vi "find and draw circles.vi"(0 "Image Src":T1, 1 "module path":path, 2 "function name":string="get_circels", 3 "initialized array":dbl[][](array[numeric]), 4 "Image Dst":T1, 5 "error in (no error)":errorcluster, 6 "session in":refnum<k35>, 7 "Run/Stop":bool, 8 "grading Thr":dbl[](array[numeric]), 9 "bias":i8=14) -> (14 "session out":refnum<k35>, 15 "circle info":dbl[][](array[numeric]), 16 "Image Out":T1, 18 "error out":errorcluster, 19 "pellet detected?":bool)   [LabVIEW 2019]
uses:
  <vilib>/vision/Image Controls.llb/IMAQ Image.ctl
  <vilib>/Utility/error.llb/DialogType.ctl
  detectedPellet.lvlib
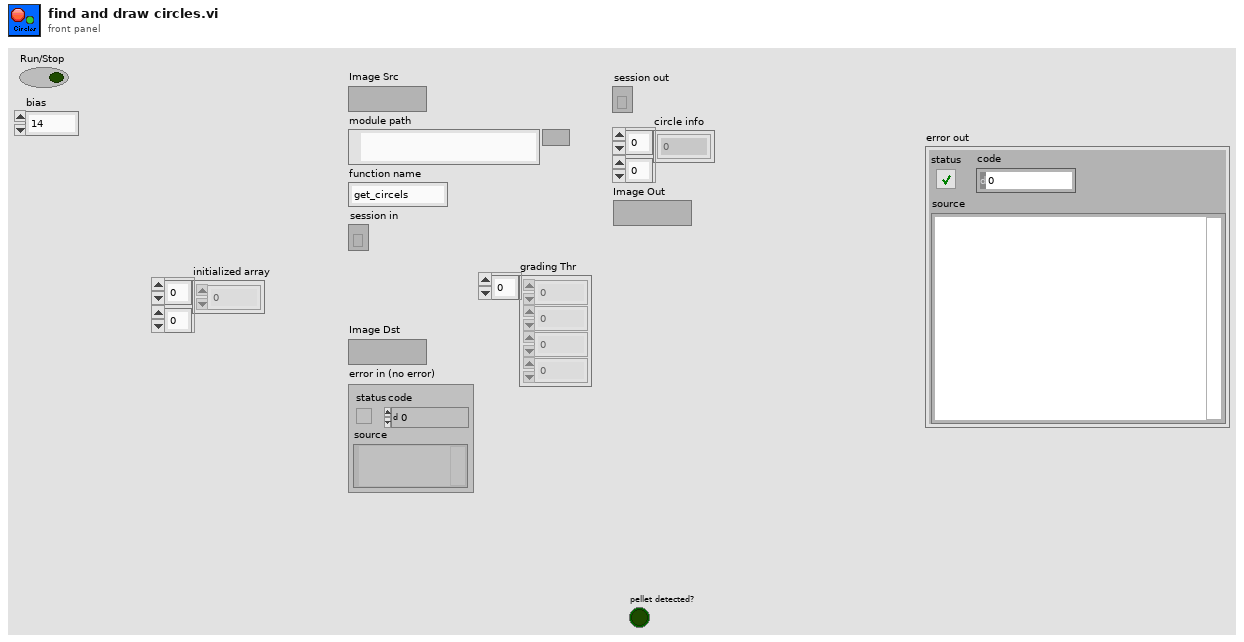
[diagram p1: front panel]
types:
  T1 = typedef "IMAQ Image.ctl" = refnum<image>
  T2 = typedef "DialogType.ctl" = u16
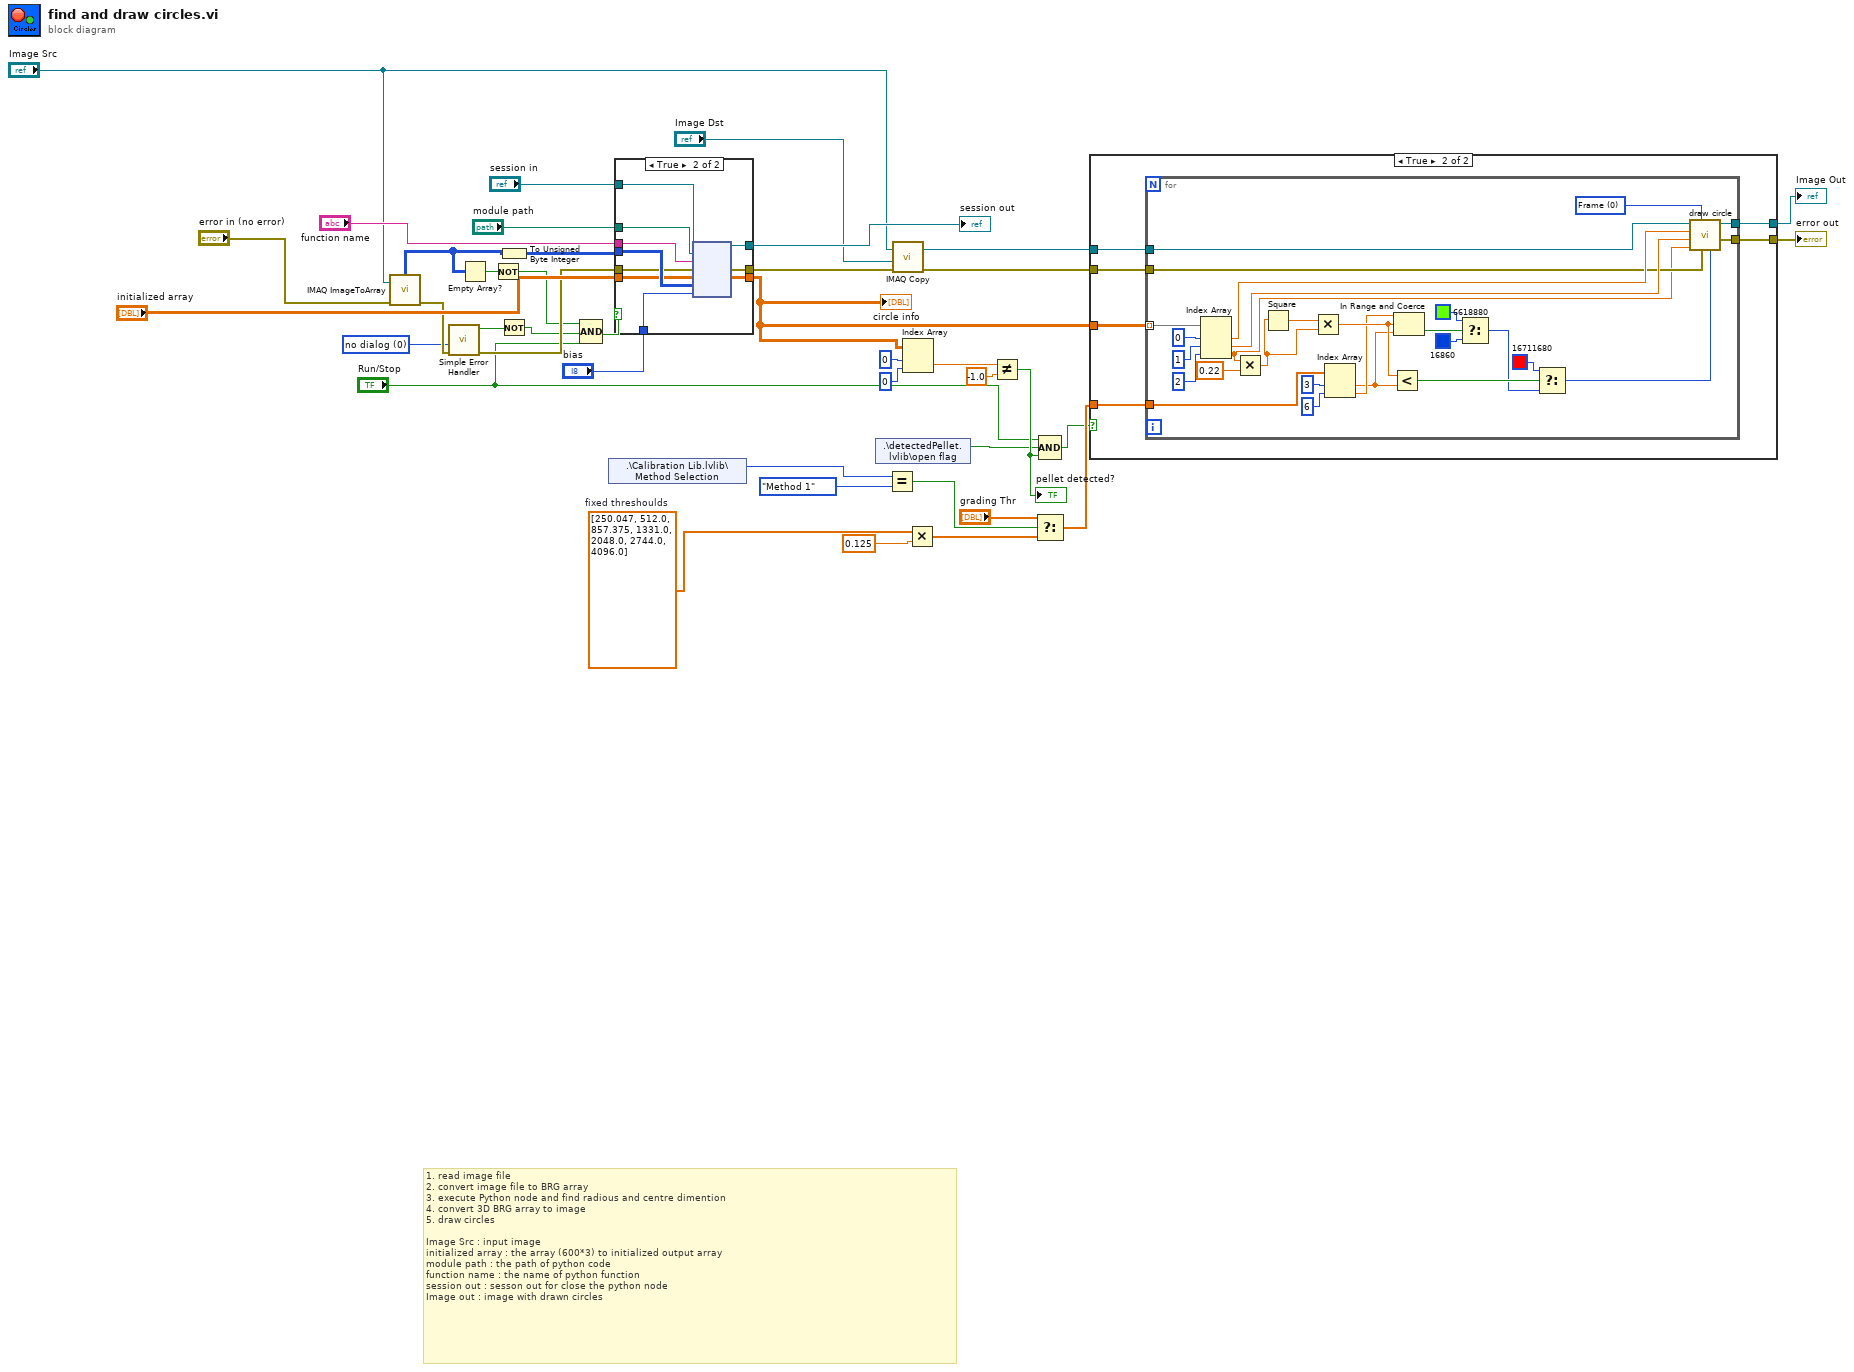
[diagram p0: block diagram]
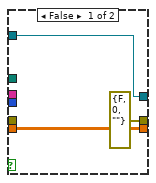
[diagram p2: hidden frame]
diagram:
  w2 = dbl[] [250.047, 512.0, 857.375, 1331.0, 2048.0, 2744.0, 4096.0]  # fixed threshoulds
  w13 = T2 0 items=["no dialog", "OK message", "continue or stop message", "OK message + warnings", "continue/stop + warnings"] ("type of dialog (OK msg:1)")
  # "1. read image file\n2. convert image file to BRG array\n3. execute Python node and find radious and centre dimention\n4. convert 3D BRG array to image\n5. draw circles\n\nImage Src : input image\ninitialized array : the array (600*3) to initialized output array \nmodule path : the path of python code\nfunction name : the name of python function \nsession out : sesson out for close the python node\nImage out : image with drawn circles"
  n1 = call "IMAQ ImageToArray"("error in (no error)"="error in (no error)", "Image"="Image Src") -> ("error out"=w15:errorcluster, "Image Pixels (U8)"=w9:u8[][])  [unwired: 2 in, 3 out]
  n2 = call <vilib>:"Simple Error Handler.vi"("type of dialog (OK msg:1)"=w13, "error in (no error)"=w15) -> ("error?"=w12:bool, "error out"=w14:errorcluster)  [unwired: 3 in, 3 out]
  n3 = Empty Array?(array=w9) -> (empty?=w8:bool)
  n4 = Not(x=w8) -> (.not. x?=w7:bool)
  n5 = To Unsigned Byte Integer(number=w9) -> (unsigned 8bit integer=w11:u8[][])
  n6 = Not(x=w12) -> (.not. x?=w6:bool)
  n7 = Compound Arithmetic op=AND(w7, w6, "Run/Stop") -> (w4:bool)
  n8 = shared-variable ".\\Calibration Lib.lvlib\\Method Selection"() -> (w24:enum32{"Method 1", "Method 2"})  [unwired: 1 in, 1 out]
  n9 = case shown="True" w4 {
    tunnel: "module path" -> [_ w54]
    tunnel: "function name" -> [_ w53]
    tunnel: w11 -> [_ w52]
    tunnel: [w44 w51] -> w38
    tunnel: "initialized array" -> [w43 w50]
    tunnel: [errorcluster {"status"=FALSE, "code"=0, "source"=""} ("function name out") w49] -> w35
    tunnel: "session in" -> [w44 w48]
    tunnel: [w43 w47] -> w1
    tunnel: w14 -> [_ w46]
    tunnel: "bias" -> [_ w45]
    frame False {
    }
    frame True {
      n10 = node(w48, w54, w53, w46, w50, w52, w45) -> (w51:refnum<k35>, w49:errorcluster, w47:dbl[][])  [unwired: 2 in, 2 out]
    }
  }
  "session out" <- w38
  "circle info" <- w1
  n11 = shared-variable ".\\detectedPellet.lvlib\\open flag"() -> (w19:bool)  [unwired: 1 in, 1 out]
  n12 = Equal?(x=w24, y=enum32{"Method 1", "Method 2"}."Method 1" ("Method Selection")) -> (x = y?=w25:bool)
  n13 = call "IMAQ Copy"("error in (no error)"=w35, "Image Dst"="Image Dst", "Image Src"="Image Src") -> ("error out"=w39:errorcluster, "Image Dst Out"=w33:T1)  [unwired: 3 in]
  n14 = Index Array(array=w1, index (row)=0, index (col)=0 ("disabled index (col)")) -> (element=w30:dbl)
  n15 = Multiply(x=w2, y=0.125) -> (x*y=w23:dbl[])
  n16 = Not Equal?(x=w30, y=-1.0) -> (x != y?=w28:bool)
  "pellet detected?" <- w28
  n17 = Select(t="grading Thr", s=w25, f=w23) -> (s? t:f=w20:dbl[])
  n18 = Compound Arithmetic op=AND("Run/Stop", w19, w28) -> (w10:bool)
  n19 = case shown="True" w10 {
    tunnel: w39 -> [w55 w62]
    tunnel: w1 -> [_ w61]
    tunnel: [w55 w60] -> w37
    tunnel: w33 -> [w56 w59]
    tunnel: [w56 w58] -> w27
    tunnel: w20 -> [_ w57]
    frame False {
    }
    frame True {
      n20 = for {
        tunnel: w59 -> [w90]
        tunnel: w61 -> [w89] mode=indexing
        tunnel: w62 -> [w82]
        tunnel: [w81] -> w60
        tunnel: [w80] -> w58
        tunnel: w57 -> [w68]
        w83 = u32 0 items=["Frame", "Fill"] ("Drawing Mode (Frame)")
        n21 = Index Array(array=w89, index #1=0 ("index"), index #2=1 ("index"), index #3=2 ("index")) -> (element #1=w85:dbl, element #2=w84:dbl, element #3=w63:dbl)
        n22 = Multiply(x=w63, y=0.22) -> (x*y=w64:dbl)
        n23 = Square(x=w64) -> (x^2=w79:dbl)
        n24 = Multiply(x=w79, y=w64) -> (x*y=w75:dbl)
        n25 = Index Array(array=w68, index #1=3 ("index"), index #2=6 ("index")) -> (element #1=w66:dbl, element #2=w67:dbl)
        n26 = Less?(x=w75, y=w66) -> (x < y?=w77:bool)
        n27 = In Range and Coerce(upper limit=w67, x=w75, lower limit=w66) -> (In Range?=w73:bool)  [unwired: 1 out]
        n28 = Select(t=u32 6618880 ("Color 2"), s=w73, f=u32 16860 ("Color 2")) -> (s? t:f=w70:u32)
        n29 = Select(t=u32 16711680 ("Color"), s=w77, f=w70) -> (s? t:f=w69:u32)
        n30 = call "draw circle.vi"("Color"=w69, "error in (no error)"=w82, "Drawing Mode (Frame)"=w83, "box size"=w63, "Y"=w84, "X"=w85, "Image In"=w90) -> ("error out"=w81:errorcluster, "Image Out"=w80:T1)  [unwired: 3 in]
      }
    }
  }
  "Image Out" <- w27
  "error out" <- w37
